vi "Modify Decal.vi"(8 "error in (no error)":errorcluster, 10 "new decal":path, 11 "ctl in":refnum<class "ctl.lvclass">) -> (0 "error out":errorcluster, 3 "ctl out":refnum<class "ctl.lvclass">)   [LabVIEW 2012, in "ctl.lvclass"]
uses:
  ctl.lvclass
  _ResManager_v86/IDClone_Resource info.ctl
  ctl.lvclass/ctl.ctl
  _ResManager_v86/IDCloneResMgr.lvlib
panel:
  out "resource info":T1 {"type" format="%.0x"}
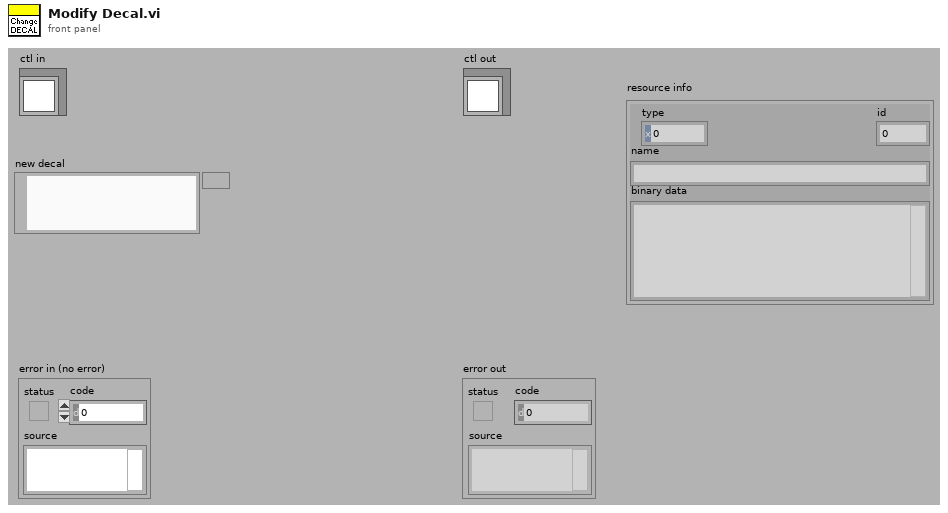
[diagram p1: front panel]
types:
  T1 = typedef "IDCloneResMgr.lvlib/IDClone_Resource info.ctl" = cluster{"type":u32, "id":i32, "name":string, "binary data":string}
  T2 = cluster{"type":u32, "id":i32, "name":string, "binary data":string}[]
  T3 = typedef "IDCloneResMgr.lvlib/ID_Resource info.ctl" = cluster{"type":u32, "id":i32, "name":string, "binary data":string}
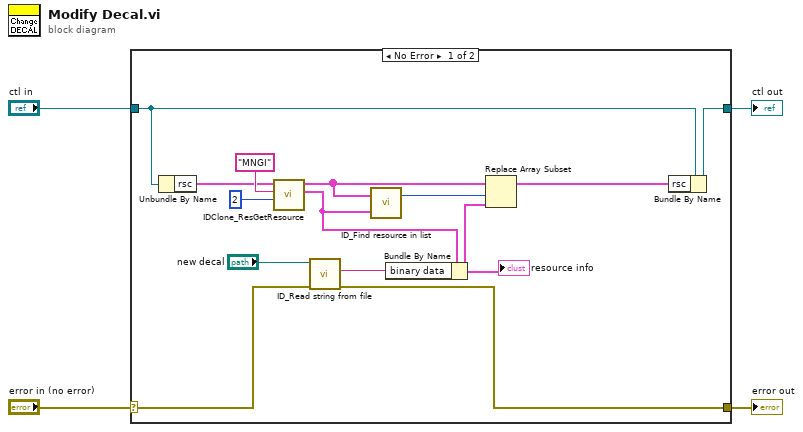
[diagram p0: block diagram]
diagram:
  n1 = case shown="No Error" "error in (no error)" {
    selector: "error in (no error)" -> [w12 w20]
    tunnel: [w11 w20] -> w3
    tunnel: [w17 w19] -> w1
    tunnel: "ctl in" -> [w18 w19]
    frame No Error {
      n2 = Unbundle By Name(w18) -> ("rsc"=w8:T2)
      n3 = call "IDClone_ResGetResource.vi"("id"=2, "type"="MNGI" ("type string"), "resources"=w8) -> ("resource info"=w6:T1, "resources"=w7:T3[])  [unwired: 1 in, 6 out]
      n4 = call "ID_Read string from file.vi"("error in (no error)"=w12, "path"="new decal") -> ("error out"=w11:errorcluster, "string"=w15:string)  [unwired: 3 in, 5 out]
      n5 = call "ID_Find resource in list.vi"("info to match"=w6, "resources"=w7) -> ("index"=w5:i32)  [unwired: 1 out]
      n6 = Bundle By Name(cluster=w6, "binary data"=w15) -> (w13:T1)
      "resource info" <- w13
      n7 = Replace Array Subset(array=w7, new element=w13, index=w5) -> (w14:T3[])
      n8 = Bundle By Name(cluster=w18, "rsc"=w14) -> (w17:refnum<class "ctl.lvclass">)
    }
    frame Error {
    }
  }
  "error out" <- w3
  "ctl out" <- w1
